vi "FindFaces.vi"() -> ()   [LabVIEW 2018]
panel:
  out "Image to process":picture
  out "Processed image":picture
  out "Error":errorcluster
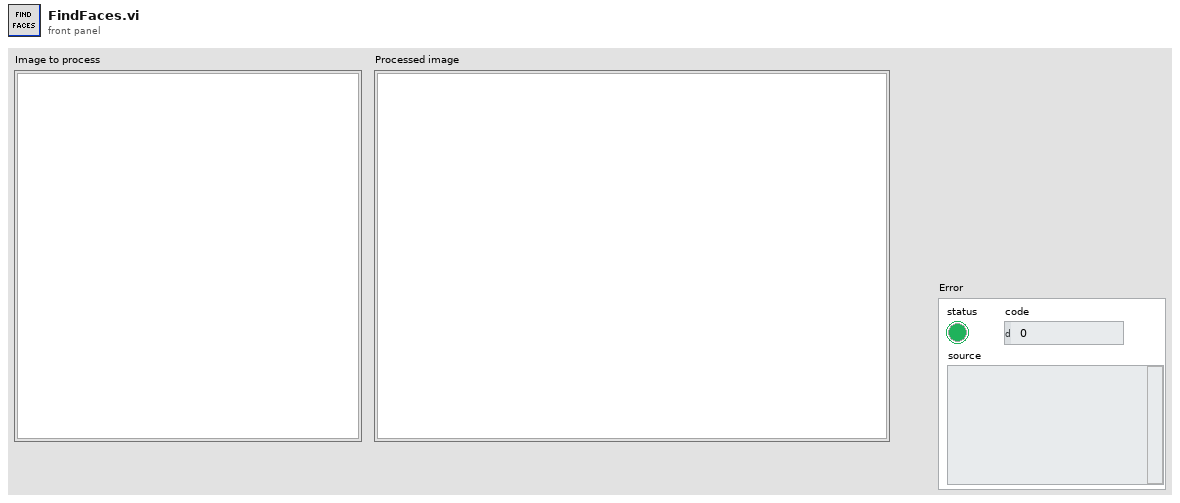
[diagram p1: front panel]
types:
  T1 = typedef "imagedata.ctl" = cluster{"image type":i32, "image depth":i32, "image":u8[], "mask":u8[], "colors":u32[], "Rectangle":cluster{"left":i16, "top":i16, "right":i16, "bottom":i16}}
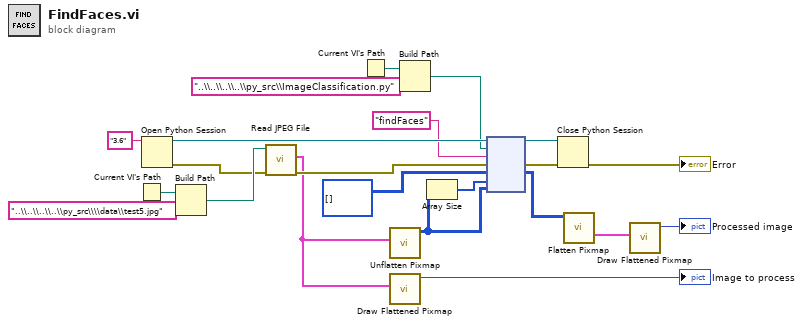
[diagram p0: block diagram]
diagram:
  n1 = Current VI's Path() -> (path=w12:path)
  n2 = Open Python Session(python version="3.6" ("Python version")) -> (session out=w22:refnum<k35>, error out=w7:errorcluster)  [unwired: 2 in]
  n3 = Build Path(base path=w12, name or relative path="..\\..\\..\\..\\py_src\\\\data\\test5.jpg") -> (appended path=w10:path)
  n4 = call <vilib>:"Read JPEG File.vi"("error in (no error)"=w7, "path to JPEG file"=w10) -> ("error out"=w6:errorcluster, "image data"=w3:T1)  [unwired: 7 in, 1 out]
  n5 = Current VI's Path() -> (path=w15:path)
  n6 = call <vilib>:"Unflatten Pixmap.vi"("image data"=w3) -> ("24-bit pixmap"=w5:u32[][])  [unwired: 4 in, 6 out]
  n7 = call <vilib>:"Draw Flattened Pixmap.vi"("image data"=w3) -> ("new picture"=→"Image to process":picture)  [unwired: 8 in]
  n8 = Build Path(base path=w15, name or relative path="..\\..\\..\\..\\py_src\\ImageClassification.py") -> (appended path=w13:path)
  n9 = Array Size(array=w5) -> (size(s)=w16:i32[])
  n10 = node(w22, w13, "findFaces" ("function name"), w6, u32[][] [], w16, w5) -> (w21:refnum<k35>, w20:errorcluster, w1:u32[][])  [unwired: 2 in, 2 out]
  n11 = Close Python Session(session in=w21, error in=w20) -> (11:→"Error":errorcluster)
  n12 = call <vilib>:"Flatten Pixmap.vi"("24-bit pixmap"=w1) -> ("image data"=w9:T1)  [unwired: 10 in]
  n13 = call <vilib>:"Draw Flattened Pixmap.vi"("image data"=w9) -> ("new picture"=→"Processed image":picture)  [unwired: 8 in]
